vi "Log.vi"(10 "Log Packet":T1, 11 "Buffered Log Sink in":refnum<class "Buffered Log Sink.lvclass">) -> (0 "error out":errorcluster, 3 "Buffered Log Sink out":refnum<class "Buffered Log Sink.lvclass">)   [LabVIEW 2018, in "MVA Framework.lvlib" / "Buffered Log Sink.lvclass"]
uses:
  Buffered Log Sink.lvclass
  Composed Log/Types/Log Level.ctl
  Composed Log/Composed Log.lvlib
  Composed Log/Types/Log Packet.ctl
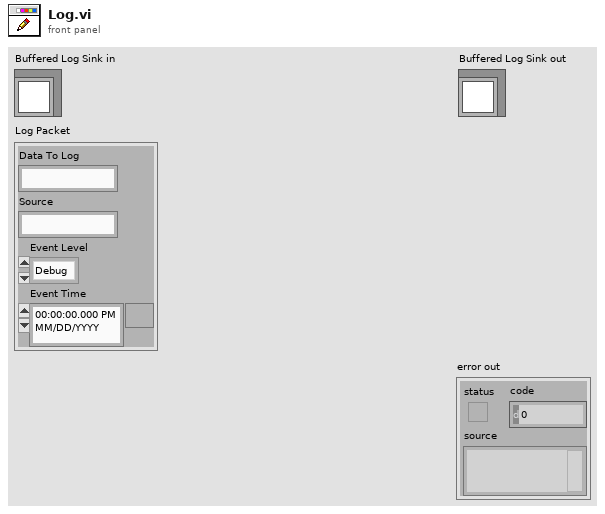
[diagram p1: front panel]
types:
  T1 = typedef "MVA Framework.lvlib/Composed Log.lvlib/Log Packet.ctl" = cluster{"Data To Log":string, "Source":string, "Event Level":T2, "Event Time":timestamp}
  T2 = typedef "MVA Framework.lvlib/Composed Log.lvlib/Log Level.ctl" = enum16{"Debug", "Info", "Warning", "Error", "Critical"}
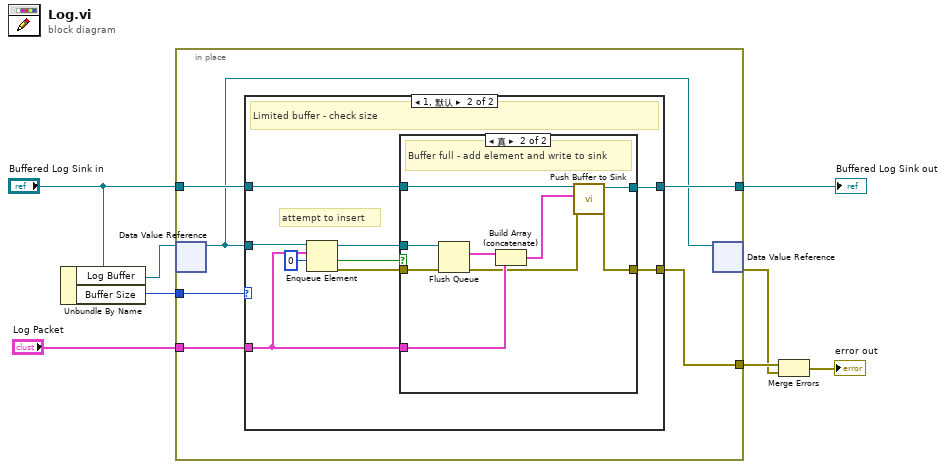
[diagram p0: block diagram]
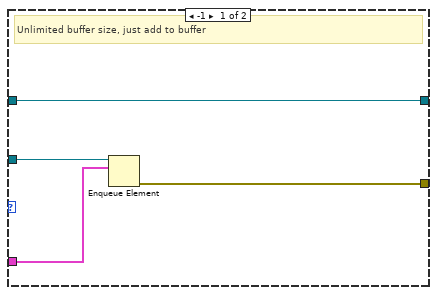
[diagram p2: hidden frame]
diagram:
  n1 = Unbundle By Name("Buffered Log Sink in") -> ("Log Buffer"=w3:refnum<data-value>, "Buffer Size"=w8:i32)
  n2 = in-place {
    in-place-border: w8 -> [w14]
    in-place-border: "Log Packet" -> [w13]
    in-place-border: [w12] -> w6
    in-place-border: "Buffered Log Sink in" -> [w11]
    in-place-border: [w10] -> w4
    n3 = in-place-dvr #1(w3) -> (w9:refnum<queue>)  [unwired: 1 out]
    n4 = case shown="1, 默认" w14 {
      tunnel: w9 -> [w18 w24]
      tunnel: w13 -> [w17 w21]
      tunnel: [w16 w25] -> w12
      tunnel: w11 -> [w15 w27]
      tunnel: [w15 w26] -> w10
      frame -1 {
        # "Unlimited buffer size, just add to buffer"
        n5 = Enqueue Element(queue=w18, element=w17) -> (error out=w16:errorcluster)  [unwired: 2 in, 2 out]
      }
      frame 1, Default {
        # "attempt to insert"
        # "Limited buffer - check size"
        n6 = Enqueue Element(queue=w24, element=w21, timeout in ms (-1)=0) -> (queue out=w22:refnum<queue>, timed out?=w19:bool, error out=w23:errorcluster)  [unwired: 1 in]
        n7 = case shown="真" w19 {
          tunnel: w27 -> [w29 w34]
          tunnel: w23 -> [w28 w37]
          tunnel: w21 -> [_ w35]
          tunnel: w22 -> [_ w38]
          tunnel: [w29 w33] -> w26
          tunnel: [w28 w30] -> w25
          frame False {
            # "Nope - we're done here"
          }
          frame True {
            # "Buffer full - add element and write to sink"
            n8 = Flush Queue(queue=w38, error in (no error)=w37) -> (remaining elements=w36:T1[], error out=w31:errorcluster)  [unwired: 1 out]
            n9 = Build Array (concatenate)(w36, w35) -> (w32:T1[])
            n10 = call "Push Buffer to Sink.vi"("error in (no error)"=w31, "Log Events"=w32, "Buffered Log Sink in"=w34) -> ("error out"=w30:errorcluster, "Buffered Log Sink out"=w33:refnum<class "Buffered Log Sink.lvclass">)  [unwired: 7 in]
          }
        }
      }
    }
    n11 = in-place-dvr #1(w9) -> (w1:errorcluster)  [unwired: 1 out]
  }
  "Buffered Log Sink out" <- w4
  n12 = Merge Errors(w6, w1) -> (→"error out":errorcluster)
